vi "TCP Server Lookup Connection Info Connection ID.vi"(8 "error in (no error)":errorcluster, 10 "connection ID":refnum<k5>, 11 "TCP Server":refnum<class "JKI TCP Server.lvclass">) -> (0 "error out":errorcluster, 3 "TCP Server out":refnum<class "JKI TCP Server.lvclass">)   [LabVIEW 2020, in "JKI TCP Server.lvclass"]
uses:
  JKI TCP Server.lvclass
  _Data Structures/TCP Server Connection Info Cluster.ctl
  JKI TCP Server.lvclass/JKI TCP Server.ctl
panel:
  out "Connection Info":T1
  # "Copyright © 2004-2008 JKI. All rights reserved.\n\nAuthor: Jim Kring [jim.kring@jameskring.com]\n\nThis library is provided \"AS IS\" ,WITHOUT WARRANTIES OR \nCONDITIONS OF ANY KIND, either express or implied.\n\nJames Kring, Inc. -- http://www.jameskring.com"
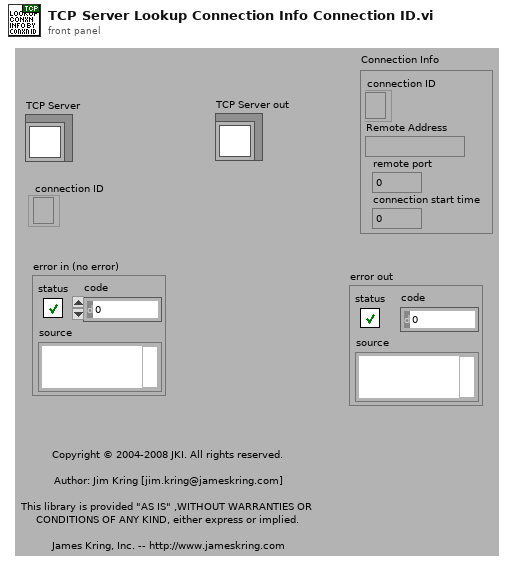
[diagram p1: front panel]
types:
  T1 = typedef "JKI TCP Server.lvclass/TCP Server Connection Info Cluster.ctl" = cluster{"connection ID":refnum<k5>, "Remote Address":string, "remote port":u16, "connection start time":u32}
  T2 = typedef "JKI TCP Server.lvclass/TCP Server Data.ctl" = cluster{"Listener Info":T3, "Connection Process VI RefNums":refnum<vi>[], "dup connection IDs (for quick search)":refnum<k5>[], "Connections":T1[], "Connection Handler VI Path":path, "Handler Is Reentrant?":bool, "TCP Handler Instance RefNums":T4[], "TCP Handler VI RefNum":T4, "No. Connections":u32, "Max Connections":u32, "server start time":u32, "Additional Data":variant}
  T3 = typedef "JKI TCP Server.lvclass/TCP Server Listener Info Cluster.ctl" = cluster{"listener ID":refnum<k5>, "net address":u32, "port":u16, "Listener Process VI Refnum":refnum<vi>}
  T4 = typedef "JKI TCP Server.lvclass/TCP Server Handler RefNum.ctl" = refnum<vi>
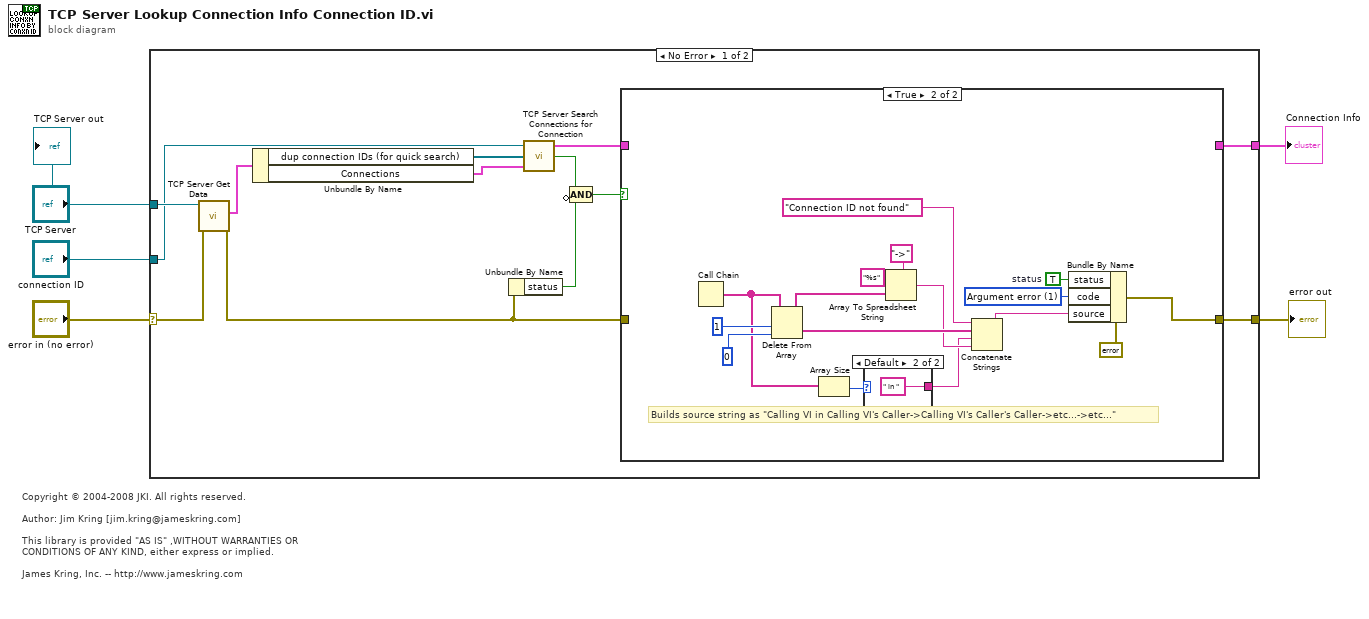
[diagram p0: block diagram]
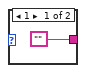
[diagram p3: hidden frame]
diagram:
  # "Copyright © 2004-2008 JKI. All rights reserved.\n\nAuthor: Jim Kring [jim.kring@jameskring.com]\n\nThis library is provided \"AS IS\" ,WITHOUT WARRANTIES OR \nCONDITIONS OF ANY KIND, either express or implied.\n\nJames Kring, Inc. -- http://www.jameskring.com"
  n1 = case shown="No Error" "error in (no error)" {
    tunnel: "TCP Server" -> [w17 _]
    tunnel: "connection ID" -> [w7 _]
    tunnel: [w8 w39] -> w4
    selector: "error in (no error)" -> [w14 w39]
    tunnel: [w10 _] -> w1
    frame No Error {
      n2 = call "TCP Server Get Data.vi"("error in (no error)"=w14, "TCP Server"=w17) -> ("error out"=w9:errorcluster, "Data out"=w18:T2)  [unwired: 7 in, 1 out]
      n3 = Unbundle By Name(w18) -> ("dup connection IDs (for quick search)"=w16:refnum<k5>[], "Connections"=w15:T1[])
      n4 = Unbundle By Name(w9) -> ("status"=w13:bool)
      n5 = call "TCP Server Search Connections for Connection.vi"("Connections"=w15, "dup connection IDs (for quick search)"=w16, "connection ID"=w7) -> ("Found?"=w6:bool, "Connection Info"=w11:T1)  [unwired: 1 out]
      n6 = Compound Arithmetic op=AND(w6, invert w13) -> (w12:bool)
      n7 = case shown="True" w12 {
        tunnel: w11 -> [w20 _]
        tunnel: [w20 _] -> w10
        tunnel: w9 -> [w19 _]
        tunnel: [w19 w35] -> w8
        frame False {
        }
        frame True {
          w30 = TRUE  # status
          w36 = 1 items=["No error", "Argument error", "Memory is full", "Out of zone", "End of file", "File already open", "Generic file I/O error", "File not found", "File permission error", "Disk is full", "Duplicate path", "Too many files open", "System feature not enabled", "Resource file not found", "Cannot add resource", "Resource not found", "Image not found", "Image memory error", "Pen does not exist", "Config type invalid", "Config token not found", "Config parse error", "Config memory error", "Bad external code format", "Bad external code offset", "External code not present", "Null window", "Destroy window error", "Null menu", "Print aborted", "Bad print record", "Print driver error", "Windows error during printing", "Memory error during printing", "Print dialog error", "Generic print error", "Invalid device refnum", "Device not found", "Device parameter error", "Device unit error", "Cannot open device", "Device call aborted", "Generic error", "Cancelled by user", "Object ID too low", "Object ID too high", "Object not in heap", "Unknown heap", "Unknown object (invalid DefProc)", "Unknown object (DefProc not in table)", "Message out of range", "Invalid (null) method", "Unknown message", "Manager call not supported", "Bad address", "Network operation in progress", "Network operation timed out", "Connection is busy", "Network attribute not supported", "Network error", "Address in use", "System out of memory", "Connection aborted", "Connection refused", "Not connected", "Already connected", "Connection closed", "Initialization error (interapplication manager)", "Bad occurrence", "Wait on unbound occurrence handler", "Occurrence queue overflow", "Datalog type conflict", "Unused", "Unrecognized type (interapplication manager)", "Memory corrupt", "Failed to make temporary DLL", "Old CIN version", "Drag socket not found", "Failed to load drop-object", "Failed to register OLE object", "Failed to release OLE object", "Format specifier type mismatch", "Unknown format specifier", "Too few format specifiers", "Too many format specifiers", "Scan failed", "Newer CIN version", "Error converting to variant", "Runtime menu error", "Password tampered", "Variant attribute not found", "Incompatible variant data type", "Event data is not available", "Event Store is not present", "Occurrence is not found", "Event Queue is not created", "Event info is not available", "Refnum passed is NULL", "Error retrieving Class GUID", "Error retrieving CoClass GUID", "Error retrieving TypeLib GUID.", "Bad built application magic bytes.", "Specific driver is different from the specific driver associated with the Logical Name.", "There is no session opened to the class driver.", "Max Error", "MAX - Error with config objects", "MAX - Error loading configuration", "MAX - Group not supported"]
          # "Builds source string as \"Calling VI in Calling VI's Caller->Calling VI's Caller's Caller->etc...->etc...\""
          n8 = Call Chain() -> (call chain=w21:string[])
          n9 = Delete From Array(array=w21, length=1 ("Length"), index=0 ("Index")) -> (deleted portion=w34:string[], array with subset deleted=w28:string[])
          n10 = Array Size(array=w21) -> (size(s)=w33:i32)
          n11 = case shown="Default" w33 {
            tunnel: ["" " in " ("Format String")] -> w23
            frame 1 {
            }
            frame Default {
            }
          }
          n12 = Array To Spreadsheet String(delimiter (Tab)="->", array=w28, 3:"%s" ("format string")) -> (spreadsheet string=w24:string)
          n13 = Concatenate Strings("Connection ID not found" ("String to Prepend to source (\"\")"), w34, w23, w24) -> (w31:string)
          n14 = Bundle By Name(cluster=errorcluster {"status"=FALSE, "code"=0, "source"=""} ("error out"), "status"=w30, "code"=w36, "source"=w31) -> (w35:errorcluster)
        }
      }
    }
    frame Error {
    }
  }
  "error out" <- w4
  "Connection Info" <- w1
  "TCP Server out" <- "TCP Server"
